vi "PostControlPlan.vi"(8 "error in (no error)":errorcluster, 10 "ControlPlan":T1, 11 "ByteGSWebAPI-V0 in":refnum<class "ByteGSWebAPI-V0.lvclass">) -> (0 "error out":errorcluster, 3 "ByteGSWebAPI-V0 out":refnum<class "ByteGSWebAPI-V0.lvclass">, 4 "body":string, 6 "headers":string)   [LabVIEW 2019, in "ByteGSWebAPI-V0.lvclass"]
uses:
  ByteGSWebAPI-V0.lvclass
  1f9a4a84-1e23-43aa-b54f-cc03f7d81dac.vi
  Cntrls/SingleControlPlan.ctl
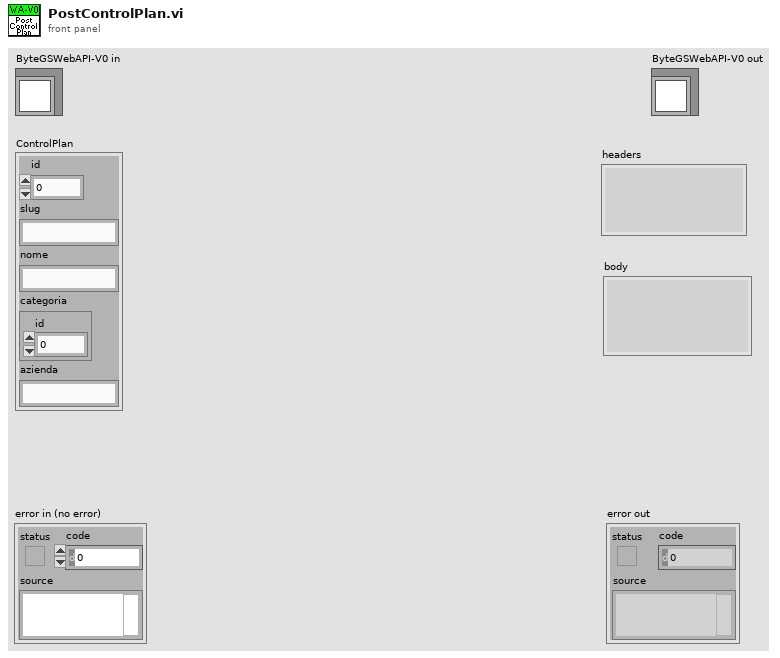
[diagram p1: front panel]
types:
  T1 = typedef "ByteGSWebAPI-V0.lvclass/SingleControlPlan.ctl" = cluster{"id":i32, "slug":string, "nome":string, "categoria":cluster{"id":i32}, "azienda":string}
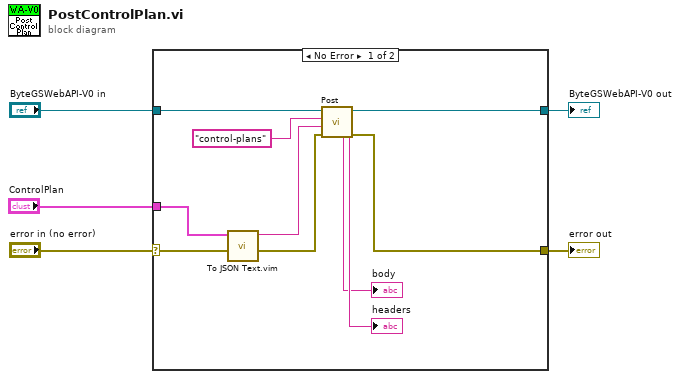
[diagram p0: block diagram]
diagram:
  n1 = case shown="No Error" "error in (no error)" {
    selector: "error in (no error)" -> [w11 w17]
    tunnel: [w7 w17] -> w4
    tunnel: [w15 w16] -> w2
    tunnel: "ByteGSWebAPI-V0 in" -> [w14 w16]
    tunnel: "ControlPlan" -> [w6 _]
    frame No Error {
      n2 = call "To JSON Text.vim"("error in (no error)"=w11, "Anything"=w6) -> ("error out"=w10:errorcluster, "<JSON>"=w9:string)  [unwired: 8 in]
      n3 = call "Post.vi"("error in (no error)"=w10, "Buffer"=w9, "Request"="control-plans", "ByteGSWebAPI-V0 in"=w14) -> ("error out"=w7:errorcluster, "Headers"=→"body":string, "Body"=→"headers":string, "ByteGSWebAPI-V0 out"=w15:refnum<class "ByteGSWebAPI-V0.lvclass">)  [unwired: 4 in]
    }
    frame Error {
    }
  }
  "error out" <- w4
  "ByteGSWebAPI-V0 out" <- w2
